vi "AddProductUnit.vi"(8 "error in":errorcluster, 9 "ProductFullName (Generic_Product)":string="Generic_Product", 10 "ProductUnitIdentifier":string, 11 "Datawarehouse in":refnum<class "Datawarehouse.lvclass">) -> (0 "error out":errorcluster, 2 "ProductUnit":refnum<class "ProductUnit.lvclass">, 3 "Datawarehouse out":refnum<class "Datawarehouse.lvclass">)   [LabVIEW 2021, in "ProligentXMLGenerator.lvlib" / "Datawarehouse.lvclass"]
doc: "Add a Product Unit.\n\nDefines a product unit. Product units are globaly unique by the combinaison of their ProductFullName and ProductUnitIdentifier properties."
uses:
  Datawarehouse.lvclass
  Datawarehouse.lvclass/Datawarehouse.ctl
  ProductUnit/ProductUnit.lvclass
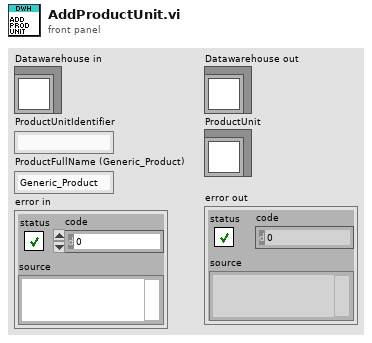
[diagram p1: front panel]
types:
  T1 = typedef "ProligentXMLGenerator.lvlib/Datawarehouse.lvclass/Data.ctl" = cluster{"DestinationFolder":path, "BaseFileName":string, "Document":refnum<k20>, "Defects":refnum<class "Defect.lvclass">[], "TopProcessRuns":refnum<class "ProcessRun.lvclass">[], "ProductUnits":refnum<class "ProductUnit.lvclass">[], "GenerationTime":refnum<class "DateTime.lvclass">, "DataSourceFingerprint":refnum<class "NonEmptyString_448.lvclass">, "IntegrationMetaData":refnum<class "NonEmptyString_2000.lvclass">, "TimeZoneInfoId":string}
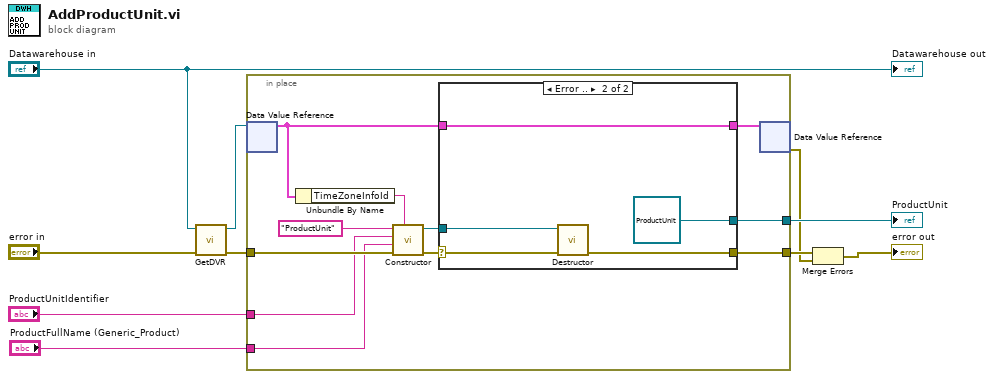
[diagram p0: block diagram]
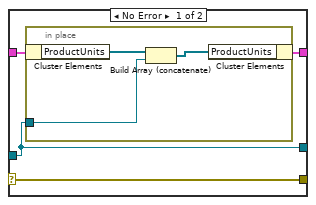
[diagram p2: hidden frame]
diagram:
  n1 = call "GetDVR.vi"("error in"="error in", "Datawarehouse"="Datawarehouse in") -> ("error out"=w4:errorcluster, "DVRReference"=w3:refnum<data-value>)  [unwired: 8 in]
  n2 = in-place "In Place Element Structure" {
    in-place-border: [w21] -> w5
    in-place-border: [w18] -> w10
    in-place-border: w4 -> [w17]
    in-place-border: "ProductUnitIdentifier" -> [w14]
    in-place-border: "ProductFullName (Generic_Product)" -> [w13]
    n3 = in-place-dvr #1(w3) -> (w12:T1)  [unwired: 1 out]
    n4 = Unbundle By Name(w12) -> ("TimeZoneInfoId"=w11:string)
    n5 = call "Constructor.vi"("TimeZoneInfoId"=w11, "error in"=w17, "ProductFullName"=w13, "ProductUnitIdentifier"=w14, "Name"="ProductUnit") -> ("error out"=w20:errorcluster, "ProductUnit out"=w19:refnum<class "ProductUnit.lvclass">)  [unwired: 5 in]
    n6 = case shown="Error .." w20 {
      selector: w20 -> [w25 w32]
      tunnel: w12 -> [w24 w33]
      tunnel: w19 -> [w22 w30]
      tunnel: [w23 w33] -> w16
      tunnel: [w25 w31] -> w21
      tunnel: [w22 refnum<class "ProductUnit.lvclass"> refnum ("TopProcessRun")] -> w18
      frame No Error {
        n7 = in-place "In Place Element Structure" {
          in-place-border: w22 -> [w26]
          n8 = in-place-cluster #2(w24) -> ("ProductUnits"=w28:refnum<class "ProductUnit.lvclass">[])
          n9 = Build Array (concatenate)(w28, w26) -> (w27:refnum<class "ProductUnit.lvclass">[])
          n10 = in-place-cluster #2("ProductUnits"=w27) -> (w23:T1)
        }
      }
      frame Error {
        n11 = call "Destructor.vi"("error in"=w32, "ProductUnit in"=w30) -> ("error out"=w31:errorcluster)  [unwired: 9 in]
      }
    }
    n12 = in-place-dvr #1(w16) -> (w2:errorcluster)  [unwired: 1 out]
  }
  "ProductUnit" <- w10
  n13 = Merge Errors(w5, w2) -> (→"error out":errorcluster)
  "Datawarehouse out" <- "Datawarehouse in"
